vi "PH_Beckhoff_PP_PU.set PSU GUI Elements to Default.vi"(0 "i ref in":refnum<vi>, 2 "PUs":T1[](array[typedef]), 5 "error in":errorcluster) -> (14 "i ref out":refnum<vi>, 19 "error out":errorcluster)   [LabVIEW 2014, in "PH_Beckhoff_PP_PU.lvlib"]
uses:
  PH_Beckhoff_PP_PU.lvlib
  PH_PP_Common/PH_PP_Common.PSU Tags.ctl
  PH_PP_Common/PH_PP_Common.PUs.ctl
  PH_Common/Names/PH_Names.Subsystems.ctl
  PH_PP_Common/PH_PP_Common.Devices.ctl
  PH_Common/PH_Common.lvlib
  PH_PP_Common/PH_PP_Common.lvlib
panel:
  in  "PSU Tags":T2
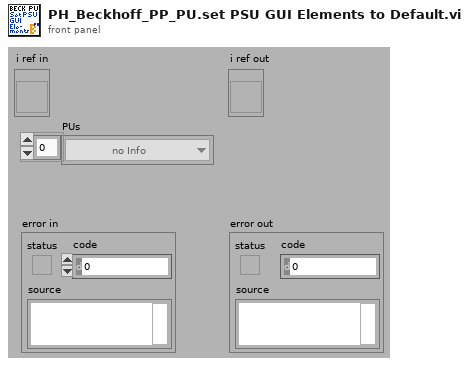
[diagram p1: front panel]
types:
  T1 = typedef "PH_PP_Common.lvlib/PH_PP_Common.PUs.ctl" = enum16{"no Info", "PA-19mm-1", "PA-19mm-2", "PA-45mm-PILC", "PA-45mm-MAIN", "MA-PU-1", "MA-PU-2", "MA-PU-3", "MA-PU-4", "MA-PU-5", "MA-PU-6", "MA-FR", "MA-PILC", "PA-45mm-DP"}
  T2 = typedef "PH_PP_Common.lvlib/PH_PP_Common.PSU Tags.ctl" = enum16{"voltage-indicator", "peak-detect", "current", "voltage", "inihibit-indicator", "end-of-charge", "HV-on-indicator", "overtemperature", "interlock-indicator", "load-fault", "sum-fault", "HV-off-indicator", "DC-ok", "inhibit", "HV-on", "interlock", "reset", "Status", "Limits"}
  T3 = typedef "PH_Common.lvlib/PH_Names.Subsystems.ctl" = enum16{"no Info", "fs-FE", "ns-FE", "PA", "MA", "MAS", "COS", "Exp-LB", "Exp-LL", "PP", "PILS"}
  T4 = typedef "PH_Beckhoff_PP_PU.lvlib/PH_Beckhoff_PP_PU.i attribute.ctl" = cluster{"HV Meas":cluster{"Input GUI Ref":refnum<vi>, "Voltage Service ID":i32, "Voltage [V]":dbl, "Quality":bool, "# in Data":i32}[], "Trigger":cluster{"Status":cluster{"GUI Ref":refnum<vi>, "Status Service ID":i32, "Status":T5}, "last shot:":cluster{"GUI Ref":refnum<vi>, "Service ID":i32, "Time":string}, "DIs":cluster{"triggered":cluster{"GUI Ref":refnum<vi>, "# in Data":i32}, "fired":cluster{"GUI Ref":refnum<vi>, "# in Data":i32}}, "GUI Ref Indicator":refnum<vi>}[], "RR":cluster{"Status":cluster{"GUI Ref":refnum<vi>, "Status Service ID":i32, "Status":T5}, "DIs":cluster{"closed":cluster{"GUI Ref":refnum<vi>, "# in Data":i32}, "open":cluster{"GUI Ref":refnum<vi>, "# in Data":i32}}, "Close":cluster{"GUI Ref":refnum<vi>, "# in Data":i32}, "GUI Ref Indicator":refnum<vi>}[], "Igni":cluster{"Status":cluster{"GUI Ref":refnum<vi>, "Status Service ID":i32, "Status":T5}, "DIs":cluster{"heating on":cluster{"GUI Ref":refnum<vi>, "# in Data":i32}, "water on":cluster{"GUI Ref":refnum<vi>, "# in Data":i32}}, "Device on":cluster{"GUI Ref":refnum<vi>, "# in Data":i32}, "GUI Ref Indicator":refnum<vi>}[], "PSU":cluster{"Status":cluster{"GUI Ref":refnum<vi>, "Status Service ID":i32, "Status":T5}, "Limit Service ID":i32, "DIs":cluster{"inhibit":cluster{"GUI Ref":refnum<vi>, "# in Data":i32}, "end of charge":cluster{"GUI Ref":refnum<vi>, "# in Data":i32}, "HV on":cluster{"GUI Ref":refnum<vi>, "# in Data":i32}, "overtemp":cluster{"GUI Ref":refnum<vi>, "# in Data":i32}, "interlock":cluster{"GUI Ref":refnum<vi>, "# in Data":i32}, "load fault":cluster{"GUI Ref":refnum<vi>, "# in Data":i32}, "sum fault":cluster{"GUI Ref":refnum<vi>, "# in Data":i32}, "HV off":cluster{"GUI Ref":refnum<vi>, "# in Data":i32}, "DC ok":cluster{"GUI Ref":refnum<vi>, "# in Data":i32}}, "AIs":cluster{"voltage":cluster{"GUI Ref":refnum<vi>, "# in Data":i32}, "current":cluster{"GUI Ref":refnum<vi>, "# in Data":i32}}, "DAs":cluster{"inhibit":cluster{"GUI Ref":refnum<vi>, "# in Data":i32}, "interlock":cluster{"GUI Ref":refnum<vi>, "# in Data":i32}, "HV on":cluster{"GUI Ref":refnum<vi>, "# in Data":i32}, "Reset":cluster{"GUI Ref":refnum<vi>, "# in Data":i32}}, "AAs":cluster{"Voltage to set":cluster{"GUI Ref":refnum<vi>, "# in Data":i32}}, "GUI Ref Indicator":refnum<vi>}[], "reconfigured":cluster{"?":bool, "GUI Ref":refnum<vi>}, "PU Rack Type":T6, "HV Meas Info":T7, "PSU Info":T8}
  T5 = typedef "PH_StatusHandler.lvlib/PH_StatusHandler.Status.ctl" = i16
  T6 = typedef "PH_Beckhoff_PP_PU.lvlib/PH_Beckhoff_PP_PU.PU Rack Type.ctl" = enum16{"no Info", "PA 19mm", "PA 45mm", "MA PU 1 and 2", "MA PU 3 and 4", "MA PU 5 and 6", "MA FR and PILC"}
  T7 = typedef "PH_Beckhoff_PP_PU.lvlib/PH_Beckhoff_PP_PU.HV Meas Info.ctl" = cluster{"Period Time [s]":dbl, "Subtractor 1 [Hz]":dbl, "Devider 1 [Hz/kV]":dbl, "Subtractor 2 [Hz]":dbl, "Devider 2 [Hz/kV]":dbl}
  T8 = typedef "PH_Beckhoff_PP_PU.lvlib/PH_Beckhoff_PP_PU.PSU Info.ctl" = cluster{"Limits 1 [V]":cluster{"Lower":dbl, "Upper":dbl}, "Limits 2 [V]":cluster{"Lower":dbl, "Upper":dbl}}
  T9 = cluster{"Status":cluster{"GUI Ref":refnum<vi>, "Status Service ID":i32, "Status":T5}, "Limit Service ID":i32, "DIs":cluster{"inhibit":cluster{"GUI Ref":refnum<vi>, "# in Data":i32}, "end of charge":cluster{"GUI Ref":refnum<vi>, "# in Data":i32}, "HV on":cluster{"GUI Ref":refnum<vi>, "# in Data":i32}, "overtemp":cluster{"GUI Ref":refnum<vi>, "# in Data":i32}, "interlock":cluster{"GUI Ref":refnum<vi>, "# in Data":i32}, "load fault":cluster{"GUI Ref":refnum<vi>, "# in Data":i32}, "sum fault":cluster{"GUI Ref":refnum<vi>, "# in Data":i32}, "HV off":cluster{"GUI Ref":refnum<vi>, "# in Data":i32}, "DC ok":cluster{"GUI Ref":refnum<vi>, "# in Data":i32}}, "AIs":cluster{"voltage":cluster{"GUI Ref":refnum<vi>, "# in Data":i32}, "current":cluster{"GUI Ref":refnum<vi>, "# in Data":i32}}, "DAs":cluster{"inhibit":cluster{"GUI Ref":refnum<vi>, "# in Data":i32}, "interlock":cluster{"GUI Ref":refnum<vi>, "# in Data":i32}, "HV on":cluster{"GUI Ref":refnum<vi>, "# in Data":i32}, "Reset":cluster{"GUI Ref":refnum<vi>, "# in Data":i32}}, "AAs":cluster{"Voltage to set":cluster{"GUI Ref":refnum<vi>, "# in Data":i32}}, "GUI Ref Indicator":refnum<vi>}[]
  T10 = typedef "PH_PP_Common.lvlib/PH_PP_Common.Devices.ctl" = enum16{"no Info", "Igni", "RR", "DumpRoss", "PSU", "Trigger", "HV-Meas", "Rods", "Chiller", "Conductivity", "Mercury"}
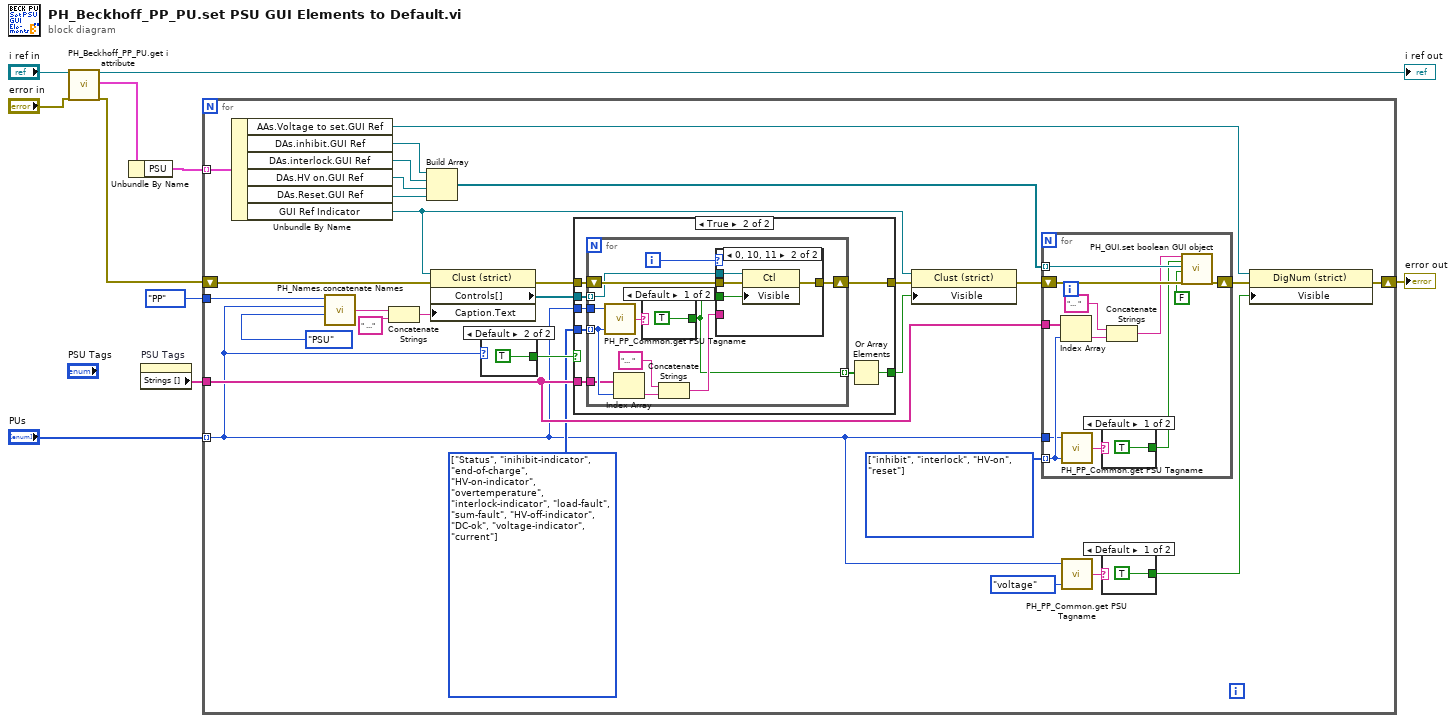
[diagram p0: block diagram]
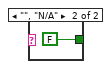
[diagram p2: hidden frame]
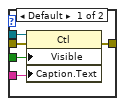
[diagram p4: hidden frame]
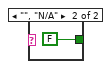
[diagram p5: hidden frame]
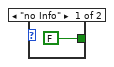
[diagram p6: hidden frame]
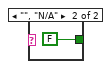
[diagram p7: hidden frame]
diagram:
  n1 = call "PH_Beckhoff_PP_PU.get i attribute.vi"("i ref in"="i ref in", "error in (no error)"="error in") -> ("i ref out"=→"i ref out":refnum<vi>, "i attribute"=w7:T4, "error out"=w5:errorcluster)  [unwired: 15 in]
  n2 = Unbundle By Name(w7) -> ("PSU"=w6:T9)
  n3 = property on="PSU Tags" class="Enum (strict)"() -> ("Strings []"=w8:string[])  [unwired: 2 in, 2 out]
  n4 = for {
    tunnel: w6 -> [w39] mode=indexing
    shift-right: [w16] -> w9
    shift-left: w5 -> [w33]
    tunnel: "PUs" -> [w12] mode=indexing
    tunnel: w8 -> [w27]
    tunnel: PH_Names.Subsystems."PP" ("Subsystem") -> [w24]
    w20 = T2[] [enum."Status", enum."inihibit-indicator", enum."end-of-charge", enum."HV-on-indicator", enum."overtemperature", enum."interlock-indicator", enum."load-fault", enum."sum-fault", enum."HV-off-indicator", enum."DC-ok", enum."voltage-indicator", enum."current"] items=["voltage-indicator", "peak-detect", "current", "voltage", "inihibit-indicator", "end-of-charge", "HV-on-indicator", "overtemperature", "interlock-indicator", "load-fault", "sum-fault", "HV-off-indicator", "DC-ok", "inhibit", "HV-on", "interlock", "reset", "Status", "Limits"]
    w18 = T2[] [enum."inhibit", enum."interlock", enum."HV-on", enum."reset"] items=["voltage-indicator", "peak-detect", "current", "voltage", "inihibit-indicator", "end-of-charge", "HV-on-indicator", "overtemperature", "interlock-indicator", "load-fault", "sum-fault", "HV-off-indicator", "DC-ok", "inhibit", "HV-on", "interlock", "reset", "Status", "Limits"]
    n5 = Unbundle By Name(w39) -> ("AAs.Voltage to set.GUI Ref"=w15:refnum<vi>, "DAs.inhibit.GUI Ref"=w37:refnum<vi>, "DAs.interlock.GUI Ref"=w36:refnum<vi>, "DAs.HV on.GUI Ref"=w35:refnum<vi>, "DAs.Reset.GUI Ref"=w21:refnum<vi>, "GUI Ref Indicator"=w23:refnum<vi>)
    n6 = call "PH_Names.concatenate Names.vi"("Devices (no info)"=PH_PP_Common.Devices."PSU", "PU (no info)"=w12, "Subsystem"=w24) -> ("Subsystem_PU_Devices_Comm Type"=w26:string)  [unwired: 1 in]
    n7 = Concatenate Strings(w26, " ..." ("string")) -> (w29:string)
    n8 = Build Array(w37, w36, w35, w21) -> (w38:refnum<vi>[])
    n9 = property class="Clust (strict)"(reference=w23, error in=w33, "Caption.Text"=w29) -> (error out=w34:errorcluster, "Controls[]"=w30:refnum<vi>[])  [unwired: 1 out]
    n10 = case shown="Default" w12 {
      tunnel: [FALSE TRUE] -> w31
      frame "no Info" {
      }
      frame Default {
      }
    }
    n11 = case shown="True" w31 {
      selector: w31 -> [w42 _]
      tunnel: w30 -> [_ w51]
      tunnel: w34 -> [w43 w50]
      tunnel: [w43 w49] -> w32
      tunnel: w20 -> [_ w48]
      tunnel: w12 -> [_ w47]
      tunnel: w27 -> [_ w46]
      tunnel: [w42 w44] -> w22
      frame False {
      }
      frame True {
        n12 = for {
          tunnel: w51 -> [w56] mode=indexing
          shift-right: [w62] -> w49
          shift-left: w50 -> [w63]
          tunnel: w47 -> [w61]
          tunnel: w48 -> [w60] mode=indexing
          tunnel: w46 -> [w59]
          tunnel: [w52] -> w45 mode=indexing
          i -> [w53]
          n13 = call "PH_PP_Common.get PSU Tagname.vi"("PSU Tag"=w60, "PU"=w61) -> ("PSU Tagname"=w58:string)  [unwired: 1 in]
          n14 = Index Array(array=w59, index=w60) -> (element=w57:string)
          n15 = case shown="Default" w58 {
            tunnel: [TRUE FALSE] -> w52
            frame Default {
            }
            frame "", "N/A" {
            }
          }
          n16 = Concatenate Strings("... " ("string"), w57) -> (w55:string)
          n17 = case shown="0, 10, 11" w53 {
            tunnel: w63 -> [w68 w72]
            tunnel: [w67 w71] -> w62
            tunnel: w52 -> [w66 w70]
            tunnel: w56 -> [w65 w69]
            tunnel: w55 -> [w64 _]
            frame Default {
              n18 = property class="Ctl"(reference=w65, error in=w68, "Visible"=w66, "Caption.Text"=w64) -> (error out=w67:errorcluster)  [unwired: 1 out]
            }
            frame 0, 10, 11 {
              n19 = property class="Ctl"(reference=w69, error in=w72, "Visible"=w70) -> (error out=w71:errorcluster)  [unwired: 1 out]
            }
          }
        }
        n20 = Or Array Elements(Boolean array=w45) -> (logical OR=w44:bool)
      }
    }
    n21 = property class="Clust (strict)"(reference=w23, error in=w32, "Visible"=w22) -> (error out=w19:errorcluster)  [unwired: 1 out]
    n22 = for {
      shift-right: [w88] -> w17
      shift-left: w19 -> [w87]
      tunnel: w38 -> [w86] mode=indexing
      tunnel: w27 -> [w82]
      tunnel: w18 -> [w78] mode=indexing
      tunnel: w12 -> [w77]
      n23 = Index Array(array=w82, index=w78) -> (element=w83:string)
      n24 = call "PH_PP_Common.get PSU Tagname.vi"("PSU Tag"=w78, "PU"=w77) -> ("PSU Tagname"=w79:string)  [unwired: 1 in]
      n25 = case shown="Default" w79 {
        tunnel: [TRUE FALSE] -> w80
        frame Default {
        }
        frame "", "N/A" {
        }
      }
      n26 = Concatenate Strings("... " ("string"), w83) -> (w84:string)
      n27 = call "PH_GUI.set boolean GUI object.vi"("Caption"=w84, "Visible (true)"=w80, "Boolean Knob GUI Ref"=w86, "Value"=FALSE, "error in (no error)"=w87) -> ("error out"=w88:errorcluster)  [unwired: 14 in]
    }
    n28 = call "PH_PP_Common.get PSU Tagname.vi"("PSU Tag"=PH_PP_Common.PSU_Tags."voltage", "PU"=w12) -> ("PSU Tagname"=w14:string)  [unwired: 1 in]
    n29 = case shown="Default" w14 {
      tunnel: [TRUE FALSE] -> w13
      frame Default {
      }
      frame "", "N/A" {
      }
    }
    n30 = property class="DigNum (strict)"(reference=w15, error in=w17, "Visible"=w13) -> (error out=w16:errorcluster)  [unwired: 1 out]
  }
  "error out" <- w9
